vi "Drive Axis Modifications.vi"(1 "Drive Info In":T1) -> (0 "Drive Info Out":T1)   [LabVIEW 2013]
uses:
  Drive Global.vi
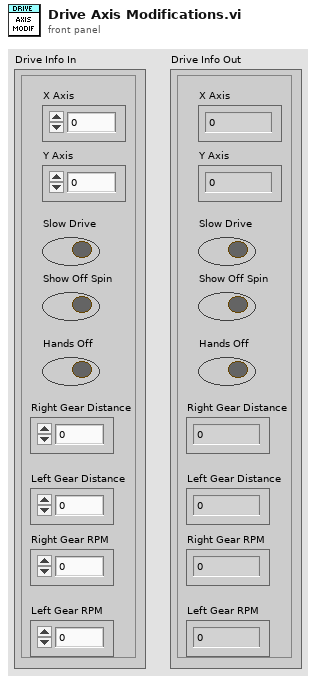
[diagram p1: front panel]
types:
  T1 = cluster{"X Axis":dbl, "Y Axis":dbl, "Slow Drive":bool, "Show Off Spin":bool, "Hands Off":bool, "Right Gear Distance":dbl, "Left Gear Distance ":dbl, "Right Gear RPM":dbl, "Left Gear RPM":dbl}
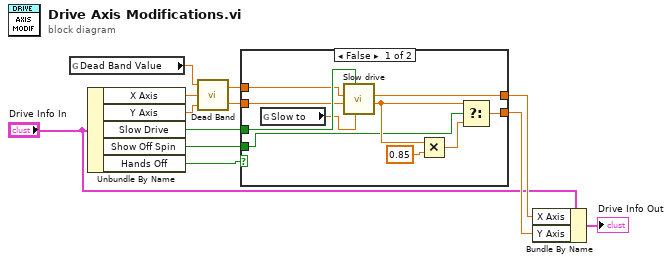
[diagram p0: block diagram]
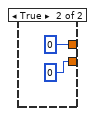
[diagram p2: hidden frame]
diagram:
  n1 = global read "Drive Global.vi" "Dead Band Value"() -> (w10:dbl)
  n2 = Unbundle By Name("Drive Info In") -> ("X Axis"=w12:dbl, "Y Axis"=w11:dbl, "Slow Drive"=w4:bool, "Show Off Spin"=w3:bool, "Hands Off"=w9:bool)
  n3 = call "Dead Band.vi"("Axis 2 In"=w11, "Axis 1 In"=w12, "Dead Band"=w10) -> ("Axis 2 Out"=w7:dbl, "Axis 1 Out"=w8:dbl)
  n4 = case shown="False" w9 {
    tunnel: w8 -> [w21 _]
    tunnel: w7 -> [w20 _]
    tunnel: [w19 0] -> w6
    tunnel: [w17 0] -> w5
    tunnel: w4 -> [w22 _]
    tunnel: w3 -> [w14 _]
    frame False {
      n5 = global read "Drive Global.vi" "Slow to"() -> (w18:dbl)
      n6 = call "Slow drive.vi"("Slow drive to"=w18, "Slow?"=w22, "Y-Axis"=w20, "X-Axis"=w21) -> ("Y - Axis out"=w16:dbl, "X-Axis out"=w19:dbl)  [unwired: 6 in]
      n7 = Multiply(x=w16, y=0.85) -> (x*y=w13:dbl)
      n8 = Select(t=w16, s=w14, f=w13) -> (s? t:f=w17:dbl)
    }
    frame True {
    }
  }
  n9 = Bundle By Name(cluster="Drive Info In", "X Axis"=w6, "Y Axis"=w5) -> (→"Drive Info Out":T1)
